vi "Get Error Message.vi"(10 "Function Name":T1, 11 "DLL Retcode":i32) -> (3 "ErrorMessage":string)   [LabVIEW 2020, in "Keyence CL-3000.lvlib"]
uses:
  Keyence CL-3000.lvlib
  enums/Function Name.ctl
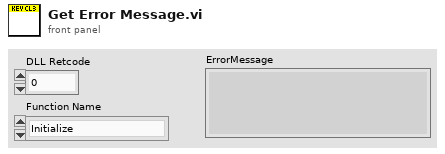
[diagram p1: front panel]
types:
  T1 = typedef "Keyence CL-3000.lvlib/Function Name.ctl" = enum16{"Initialize", "Close", "CL3IF_GetMeasurementData", "CL3IF_GetTrendIndex", "CL3IF_GetTrendData", "CL3IF_GetStorageIndex", "CL3IF_GetStorageData", "CL3IF_AutoZeroMulti", "CL3IF_AutoZeroGroup", "CL3IF_TimingMulti", "CL3IF_TimingGroup", "CL3IF_ResetMulti", "CL3IF_ResetGroup", "CL3IF_LightControl", "CL3IF_MeasurementControl", "CL3IF_SwitchProgram", "CL3IF_GetProgramNo", "CL3IF_StartStorage", "CL3IF_StopStorage", "CL3IF_ClearStorageData", "CL3IF_GetPulseCount", "CL3IF_ResetPulseCount", "CL3IF_GetLightWaveform"}
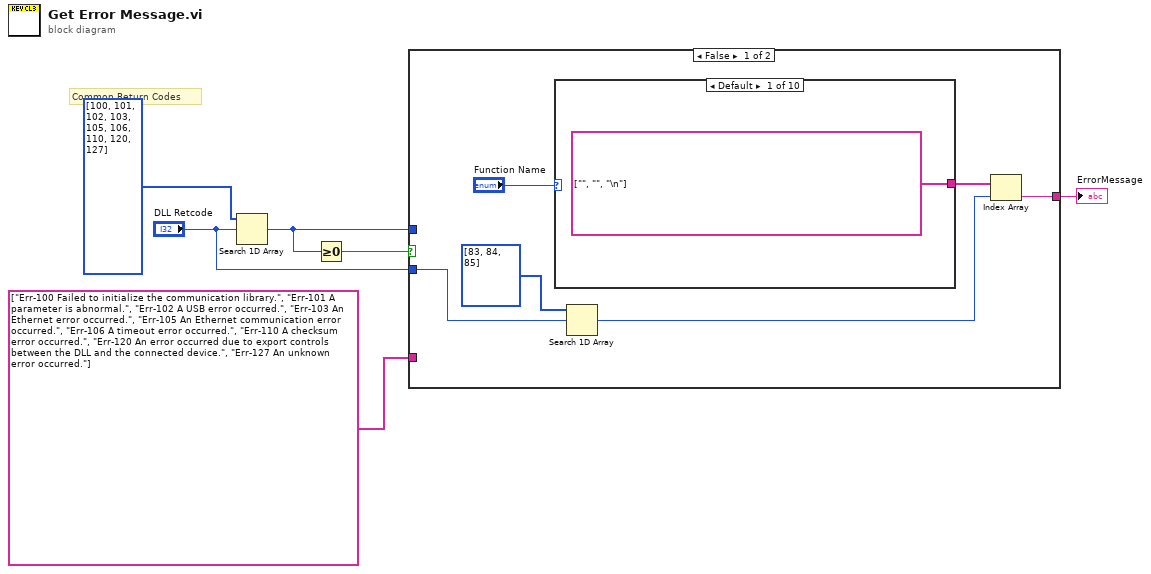
[diagram p0: block diagram]
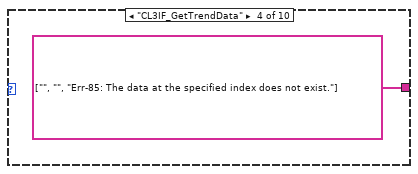
[diagram p4: hidden frame]
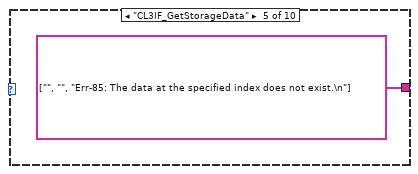
[diagram p5: hidden frame]
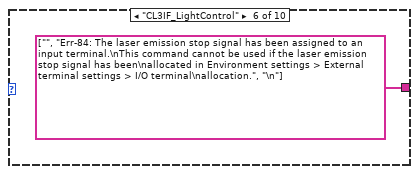
[diagram p6: hidden frame]
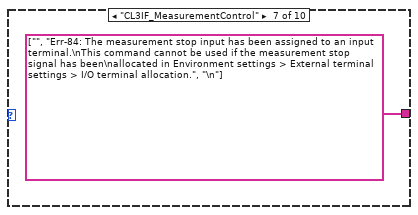
[diagram p7: hidden frame]
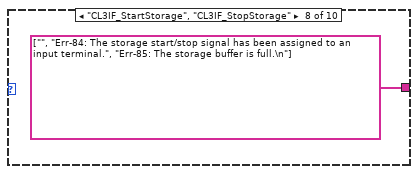
[diagram p8: hidden frame]
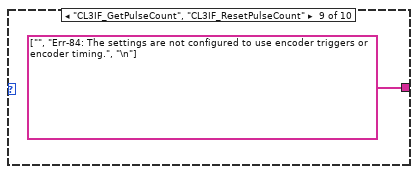
[diagram p9: hidden frame]
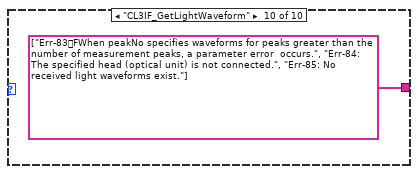
[diagram p10: hidden frame]
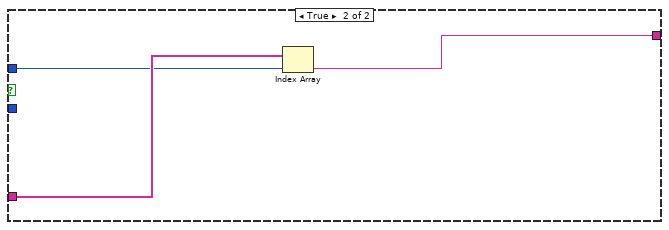
[diagram p11: hidden frame]
diagram:
  # "Common Return Codes"
  n1 = Search 1D Array(1D array=i32[] [100, 101, 102, 103, 105, 106, 110, 120, 127], element="DLL Retcode") -> (index of element=w3:i32)  [unwired: 1 in]
  n2 = Greater Or Equal To 0?(x=w3) -> (x >= 0?=w5:bool)
  n3 = case shown="False" w5 {
    tunnel: string[] ["Err-100 Failed to initialize the communication library.", "Err-101 A parameter is abnormal.", "Err-102 A USB error occurred.", "Err-103 An Ethernet error occurred.", "Err-105 An Ethernet communication error occurred.", "Err-106 A timeout error occurred.", "Err-110 A checksum error occurred.", "Err-120 An error occurred due to export controls between the DLL and the connected device.", "Err-127 An unknown error occurred."] -> [_ w23]
    tunnel: w3 -> [_ w22]
    tunnel: [w7 w21] -> w2
    tunnel: "DLL Retcode" -> [w11 _]
    frame False {
      n4 = case shown="Default" "Function Name" {
        tunnel: [string[] ["", "", "\n"] _ _ string[] ["", "", "Err-85: The data at the specified index does not exist."] string[] ["", "", "Err-85: The data at the specified index does not exist.\n"] string[] ["", "Err-84: The laser emission stop signal has been assigned to an input terminal.\nThis command cannot be used if the laser emission stop signal has been\nallocated in Environment settings > External terminal settings > I/O terminal\nallocation.", "\n"] string[] ["", "Err-84: The measurement stop input has been assigned to an input terminal.\nThis command cannot be used if the measurement stop signal has been\nallocated in Environment settings > External terminal settings > I/O terminal allocation.", "\n"] string[] ["", "Err-84: The storage start/stop signal has been assigned to an input terminal.", "Err-85: The storage buffer is full.\n"] string[] ["", "Err-84: The settings are not configured to use encoder triggers or encoder timing.", "\n"] string[] ["Err-83FWhen peakNo specifies waveforms for peaks greater than the number of measurement peaks, a parameter error  occurs.", "Err-84: The specified head (optical unit) is not connected.", "Err-85: No received light waveforms exist."]] -> w9
        frame Default {
        }
        frame "Initialize" {
        }
        frame "Close" {
        }
        frame "CL3IF_GetTrendData" {
        }
        frame "CL3IF_GetStorageData" {
        }
        frame "CL3IF_LightControl" {
        }
        frame "CL3IF_MeasurementControl" {
        }
        frame "CL3IF_StartStorage", "CL3IF_StopStorage" {
        }
        frame "CL3IF_GetPulseCount", "CL3IF_ResetPulseCount" {
        }
        frame "CL3IF_GetLightWaveform" {
        }
      }
      n5 = Search 1D Array(1D array=i32[] [83, 84, 85], element=w11) -> (index of element=w8:i32)  [unwired: 1 in]
      n6 = Index Array(array=w9, index=w8) -> (element=w7:string)
    }
    frame True {
      n7 = Index Array(array=w23, index=w22) -> (element=w21:string)
    }
  }
  "ErrorMessage" <- w2
